vi "Clapper.vi"(7 "State":T4=enum."Out", 8 "Error in":errorcluster, 10 "Plugged":T1={"DevStatus"={"status"=FALSE, "code"=0, "source"=""}, "Solenoid Module"=enum."Solenoid Module 1", "Forward Solenoid Channel"=enum."Invalid", "Reverse Solenoid Channel"=enum."Invalid"}, 11 "Open":T1={"DevStatus"={"status"=FALSE, "code"=0, "source"=""}, "Solenoid Module"=enum."Solenoid Module 1", "Forward Solenoid Channel"=enum."Invalid", "Reverse Solenoid Channel"=enum."Invalid"}) -> (0 "Error out":errorcluster)   [LabVIEW 2013]
doc: "VI for the clapper double solenoid. It has the following actions:\n-Init: take a reference to a double solenoid and store it in a shift register so that it does not need to be passed in again.\n-In: sets the cylinder to the in position.\n-Middle: set the cylinder to the middle position.\n-Out: set the cylinder to the out position."
uses:
  <vilib>/Rock Robotics/WPI/Solenoid/WPI_SolenoidDevRef.ctl
  <vilib>/Rock Robotics/SystemInterfaces/Typedef/FPGA_TypedefSolenoidModule.ctl
  <vilib>/Rock Robotics/WPI/Solenoid/WPI_SolenoidChannel.ctl
  DoubleSolenoidAction.ctl
  <vilib>/Rock Robotics/WPI/Solenoid/WPI_SolenoidValue.ctl
  <vilib>/Rock Robotics/WPI/Solenoid/WPI_SolenoidSetEnum.vi
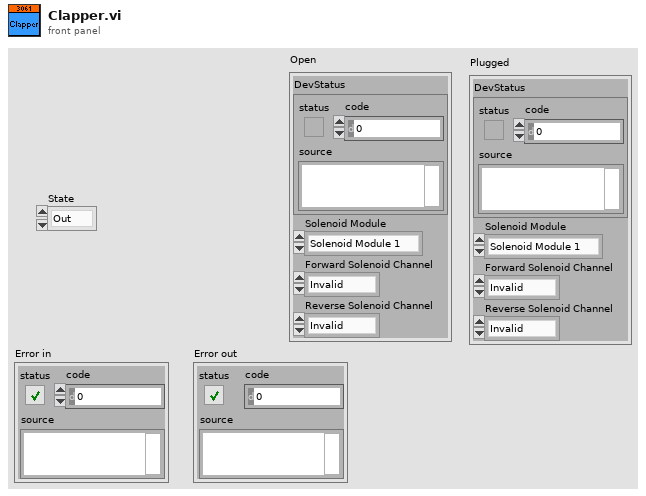
[diagram p1: front panel]
types:
  T1 = typedef "WPI_SolenoidDevRef.ctl" = cluster{"DevStatus":errorcluster, "Solenoid Module":T2, "Forward Solenoid Channel":T3, "Reverse Solenoid Channel":T3}
  T2 = typedef "FPGA_TypedefSolenoidModule.ctl" = enum16{"Solenoid Module 1", "Solenoid Module 2"}
  T3 = typedef "WPI_SolenoidChannel.ctl" = enum8{"Solenoid 1", "Solenoid 2", "Solenoid 3", "Solenoid 4", "Solenoid 5", "Solenoid 6", "Solenoid 7", "Solenoid 8", "Invalid"}
  T4 = typedef "DoubleSolenoidAction.ctl" = enum16{"Init", "Middle", "In", "Out"}
  T5 = typedef "WPI_SolenoidValue.ctl" = enum16{"Off", "On", "Forward", "Reverse"}
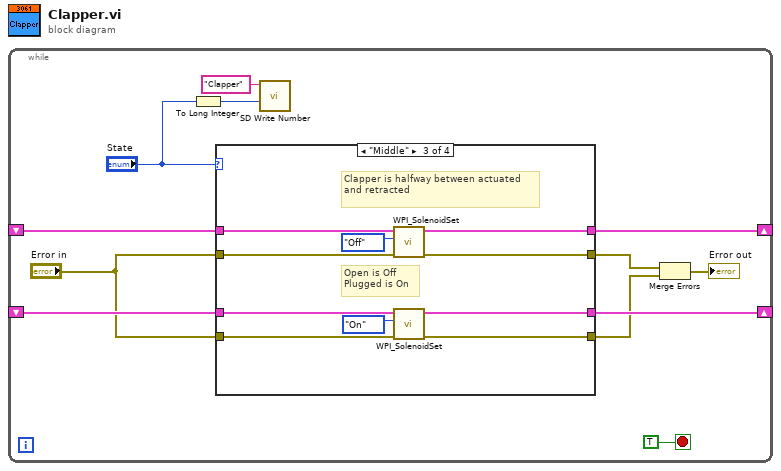
[diagram p0: block diagram]
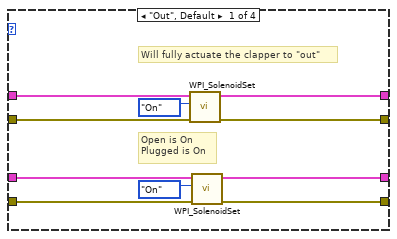
[diagram p2: hidden frame]
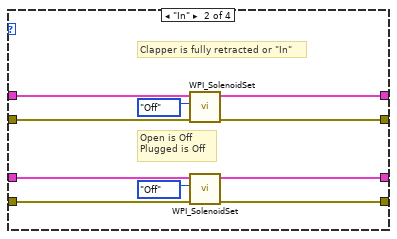
[diagram p3: hidden frame]
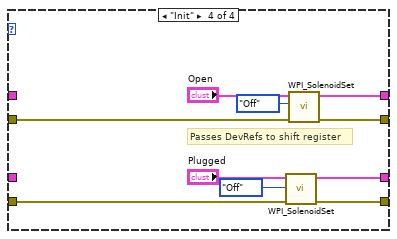
[diagram p4: hidden frame]
diagram:
  n1 = while {
    shift-right: [w11] -> _
    shift-left: _ -> [w10]
    shift-right: [w8] -> _
    shift-left: _ -> [w7]
    stop <- TRUE stop-if-true
    n2 = To Long Integer(number="State") -> (32bit integer=w3:i32)
    n3 = case shown="\"Middle\"" "State" {
      tunnel: [w22 w32 w42 w51] -> w11
      tunnel: w10 -> [w20 w30 w41 _]
      tunnel: "Error in" -> [w19 w29 w40 w49]
      tunnel: [w18 w28 w39 w48] -> w9
      tunnel: [w16 w26 w36 w46] -> w8
      tunnel: w7 -> [w17 w27 w37 _]
      tunnel: "Error in" -> [w14 w25 w34 w45]
      tunnel: [w13 w24 w35 w44] -> w4
      frame "Out", Default {
        # "Open is On\nPlugged is On"
        # "Will fully actuate the clapper to \"out\""
        n4 = call-poly <vilib>:"WPI_SolenoidSet.vi"("error in (no error)"=w19, "Value"=WPI_SolenoidValue."On", "SolenoidDevRef"=w20) -> ("error out"=w18:errorcluster, "SolenoidDevRef"=w22:T1)  [unwired: 7 in]
        n5 = call-poly <vilib>:"WPI_SolenoidSet.vi"("error in (no error)"=w14, "Value"=WPI_SolenoidValue."On", "SolenoidDevRef"=w17) -> ("error out"=w13:errorcluster, "SolenoidDevRef"=w16:T1)  [unwired: 7 in]
      }
      frame "In" {
        # "Open is Off\nPlugged is Off"
        # "Clapper is fully retracted or \"In\""
        n6 = call-poly <vilib>:"WPI_SolenoidSet.vi"("error in (no error)"=w29, "Value"=WPI_SolenoidValue."Off", "SolenoidDevRef"=w30) -> ("error out"=w28:errorcluster, "SolenoidDevRef"=w32:T1)  [unwired: 7 in]
        n7 = call-poly <vilib>:"WPI_SolenoidSet.vi"("error in (no error)"=w25, "Value"=WPI_SolenoidValue."Off", "SolenoidDevRef"=w27) -> ("error out"=w24:errorcluster, "SolenoidDevRef"=w26:T1)  [unwired: 7 in]
      }
      frame "Middle" {
        # "Open is Off\nPlugged is On"
        # "Clapper is halfway between actuated and retracted"
        n8 = call-poly <vilib>:"WPI_SolenoidSet.vi"("error in (no error)"=w40, "Value"=WPI_SolenoidValue."Off", "SolenoidDevRef"=w41) -> ("error out"=w39:errorcluster, "SolenoidDevRef"=w42:T1)  [unwired: 7 in]
        n9 = call-poly <vilib>:"WPI_SolenoidSet.vi"("error in (no error)"=w34, "Value"=WPI_SolenoidValue."On", "SolenoidDevRef"=w37) -> ("error out"=w35:errorcluster, "SolenoidDevRef"=w36:T1)  [unwired: 7 in]
      }
      frame "Init" {
        # "Passes DevRefs to shift register"
        n10 = call-poly <vilib>:"WPI_SolenoidSet.vi"("error in (no error)"=w45, "Value"=WPI_SolenoidValue."Off", "SolenoidDevRef"="Plugged") -> ("error out"=w44:errorcluster, "SolenoidDevRef"=w46:T1)  [unwired: 7 in]
        n11 = call-poly <vilib>:"WPI_SolenoidSet.vi"("error in (no error)"=w49, "Value"=WPI_SolenoidValue."Off", "SolenoidDevRef"="Open") -> ("error out"=w48:errorcluster, "SolenoidDevRef"=w51:T1)  [unwired: 7 in]
      }
    }
    n12 = call <vilib>:"SD Write Number.vi"("Numeric"=w3, "Name"="Clapper") -> ()  [unwired: 8 in, 2 out]
    n13 = Merge Errors(w9, w4) -> (→"Error out":errorcluster)
  }
